vi "Restart time.vi"(8 "error in (no error)":errorcluster, 11 "Elevator Controller in":refnum<class "Elevator Controller.lvclass">) -> (0 "error out":errorcluster, 3 "Elevator Controller out":refnum<class "Elevator Controller.lvclass">)   [LabVIEW 2019, in "Elevator Controller.lvlib" / "Elevator Controller.lvclass"]
uses:
  Elevator Controller.lvclass
  Elevator Controller.lvclass/Elevator Controller.ctl
  Sim Display Console Actor/Sim Display Console Actor Messages/Write Timing Msg/Write Timing Msg.lvclass/Write Timing Msg.ctl
  <vilib>/ActorFramework/Message Enqueuer/Message Enqueuer.lvclass/Message Enqueuer.ctl
  <vilib>/ActorFramework/Message Enqueuer/Enqueue.vi
  Sim Display Console Actor/Sim Display Console Actor Messages/Write Timing Msg/Write Timing Msg.lvclass
  C:/Program Files (x86)/National Instruments/LabVIEW 2019/vi.lib/ActorFramework/Message/Message.lvclass
  <vilib>/ActorFramework/Message Priority Queue/Priority Enqueue.vi
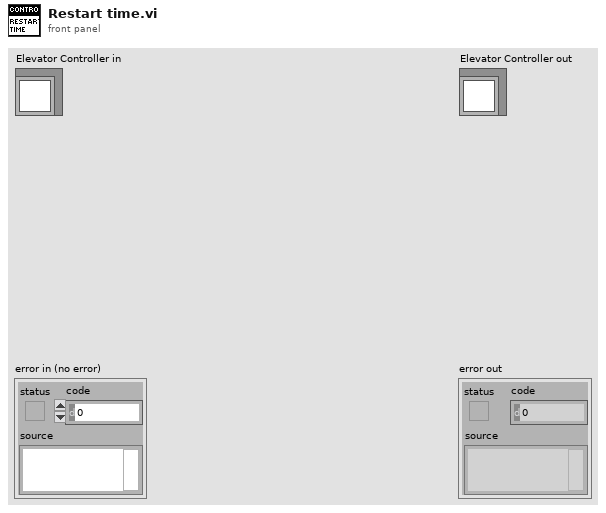
[diagram p1: front panel]
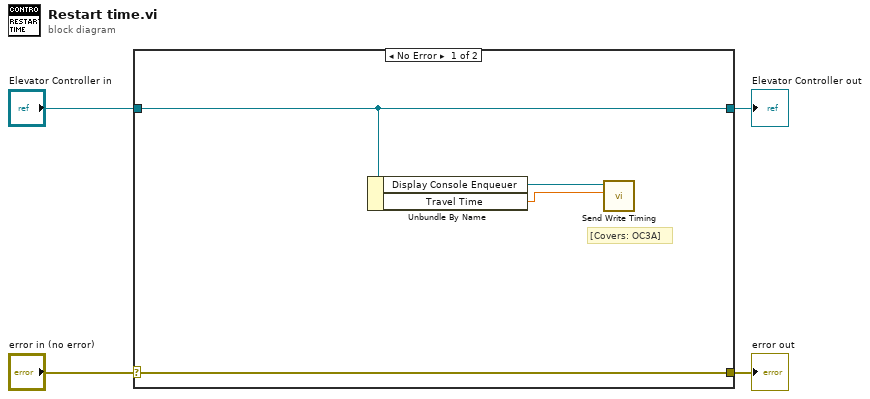
[diagram p0: block diagram]
diagram:
  n1 = case shown="No Error" "error in (no error)" {
    selector: "error in (no error)" -> [w8 w10]
    tunnel: [w8 w10] -> w3
    tunnel: [w7 w9] -> w1
    tunnel: "Elevator Controller in" -> [w7 w9]
    frame No Error {
      # "[Covers: OC3A]"
      n2 = Unbundle By Name(w7) -> ("Display Console Enqueuer"=w6:refnum<class "Message Enqueuer.lvclass">, "Travel Time"=w5:dbl)
      n3 = call "Send Write Timing.vi"("timing"=w5, "Message Enqueuer"=w6) -> ()  [unwired: 8 in, 2 out]
    }
    frame Error {
    }
  }
  "error out" <- w3
  "Elevator Controller out" <- w1
